vi "NaN 与任何数都不相等，包括它自己.vi"() -> ()   [LabVIEW 2020]
panel:
  out "NaN 只能使用“不是一个数字/路径/引用”函数来检查":bool
  out "NaN等于NaN吗？=False":bool
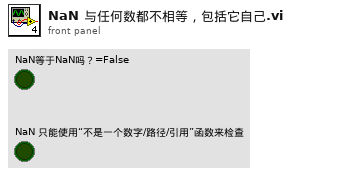
[diagram p1: front panel]
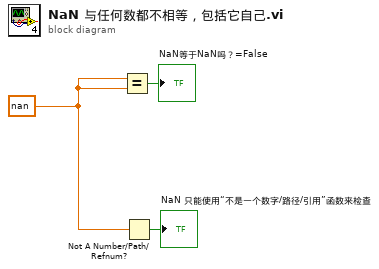
[diagram p0: block diagram]
diagram:
  w3 = nan
  n1 = Equal?(x=w3, y=w3) -> (x = y?=→"NaN等于NaN吗？=False":bool)
  n2 = Not A Number/Path/Refnum?(number/path/refnum=w3) -> (NaN/Path/Refnum?=→"NaN 只能使用“不是一个数字/路径/引用”函数来检查":bool)
